vi "NI-9213_SoftPanel.vi"(3 "NI-9213 in Slot:":string="1") -> ()   [LabVIEW 2016]
uses:
  HelperSubVIs/GlobalControlVariables.vi
  <vilib>/Utility/TradDaqScaling.llb/Convert Thermocouple Reading (scaler).vi
panel:
  in  "Temperature Units":string(combo)="0"
  in  "TC 15 Type":string(combo)="0"
  in  "TC 14 Type":string(combo)="0"
  in  "TC 13 Type":string(combo)="0"
  in  "TC 12 Type":string(combo)="0"
  in  "TC 11 Type":string(combo)="0"
  in  "TC 10 Type":string(combo)="0"
  in  "TC 09 Type":string(combo)="0"
  in  "TC 08 Type":string(combo)="0"
  in  "TC 07 Type":string(combo)="0"
  in  "TC 06 Type":string(combo)="0"
  in  "TC 05 Type":string(combo)="0"
  in  "TC 04 Type":string(combo)="0"
  in  "TC 03 Type":string(combo)="0"
  in  "TC 02 Type":string(combo)="0"
  in  "TC 01 Type":string(combo)="0"
  in  "TC 00 Type":string(combo)="0"
  out "AI Values":sgl[](array[numeric])
  out "ExitModule":bool=TRUE
  out "TC 07":sgl
  out "TC 06":sgl
  out "TC 05":sgl
  out "TC 04":sgl
  out "TC 03":sgl
  out "TC 02":sgl
  out "TC 01":sgl
  out "TC 00":sgl
  out "TC 15":sgl min=0 max=5
  out "TC 14":sgl min=0 max=5
  out "TC 13":sgl min=0 max=5
  out "TC 12":sgl min=0 max=5
  out "TC 11":sgl min=0 max=5
  out "TC 10":sgl min=0 max=5
  out "TC 09":sgl min=0 max=5
  out "TC 08":sgl min=0 max=5
  in  "ExitButton":bool
  # "Thermocouple Type"
  # "Thermocouple Value"
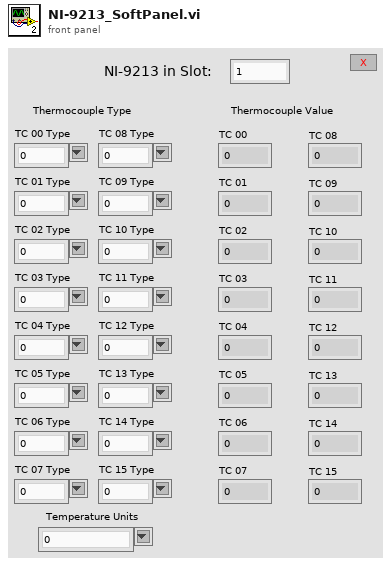
[diagram p1: front panel]
types:
  T1 = cluster{"[0]":sgl, "[1]":sgl, "[2]":sgl, "[3]":sgl, "[4]":sgl, "[5]":sgl, "[6]":sgl, "[7]":sgl, "[8]":sgl, "[9]":sgl, "[10]":sgl, "[11]":sgl, "[12]":sgl, "[13]":sgl, "[14]":sgl, "[15]":sgl}
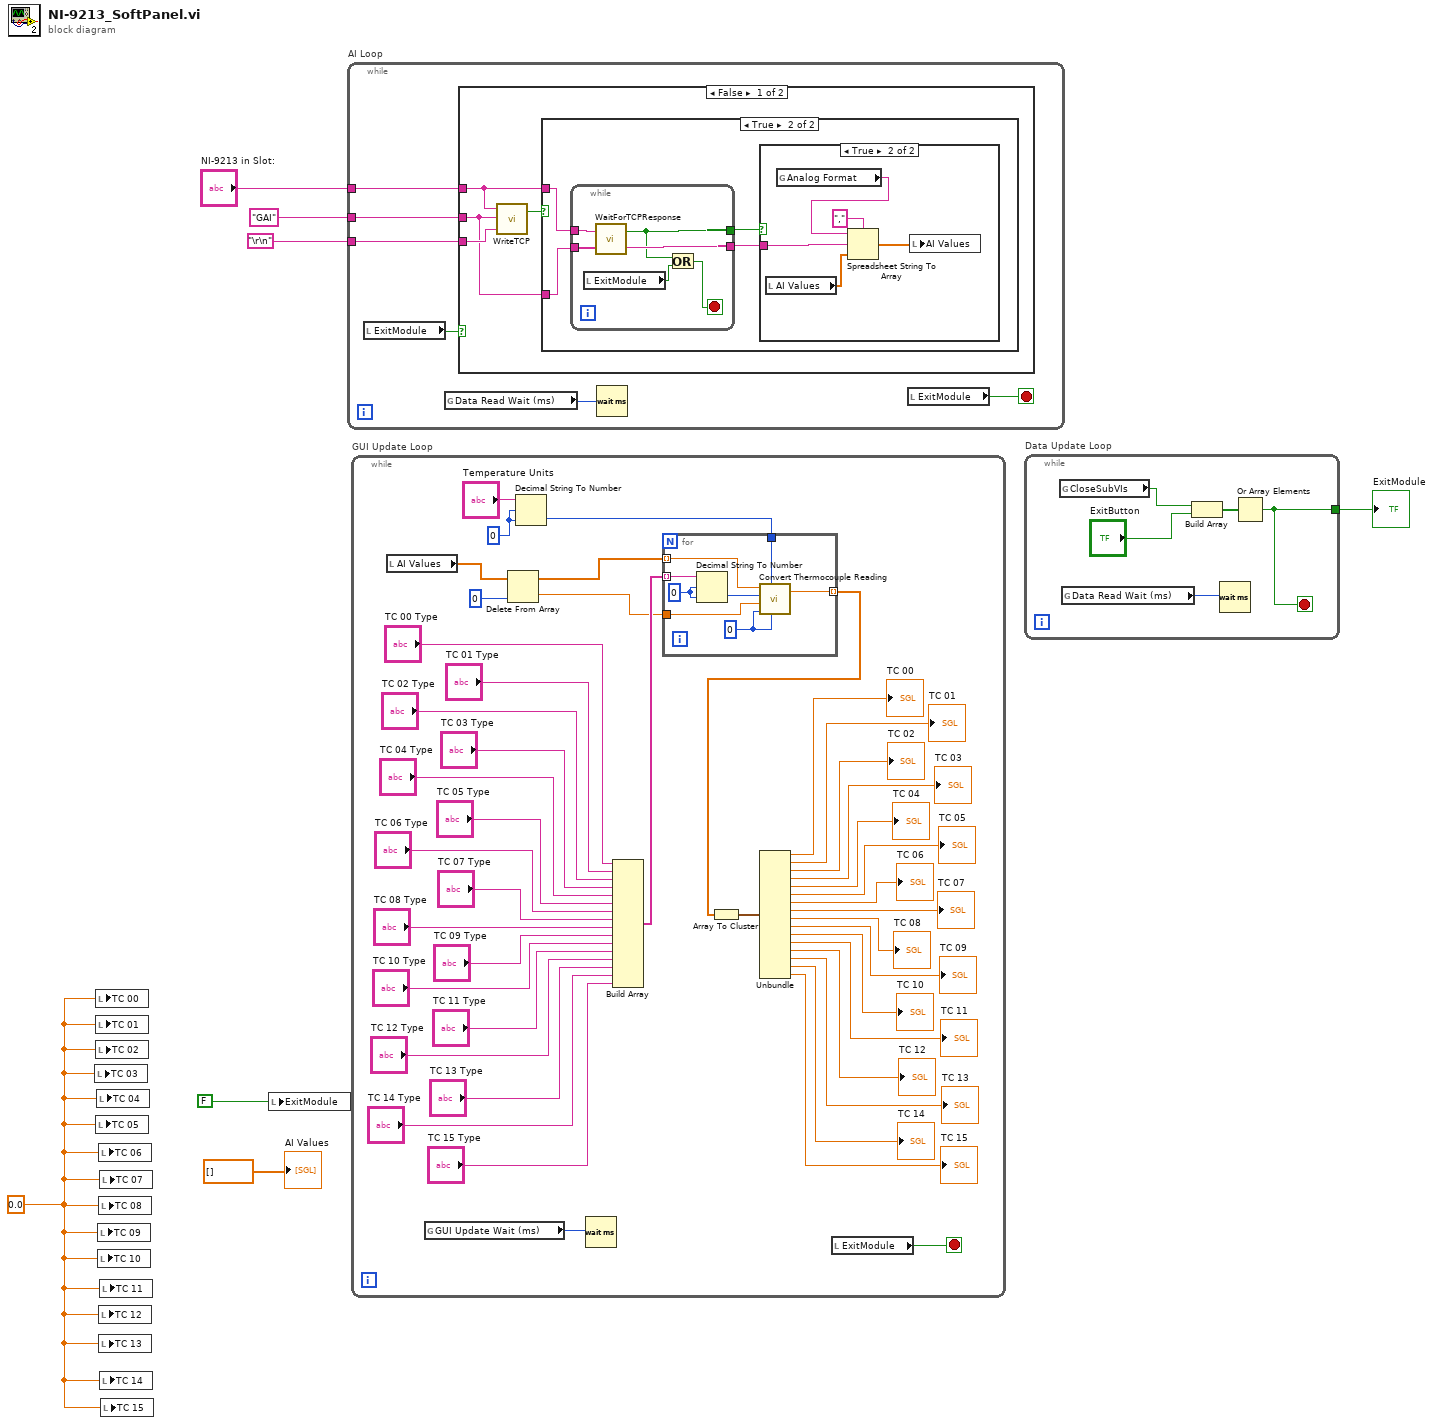
[diagram p0: block diagram]
diagram:
  w2 = 0.0
  n1 = local write "TC 03"(w2) -> ()
  n2 = local write "TC 00"(w2) -> ()
  n3 = local write "TC 01"(w2) -> ()
  n4 = local write "TC 02"(w2) -> ()
  n5 = local write "TC 05"(w2) -> ()
  n6 = local write "TC 04"(w2) -> ()
  n7 = local write "TC 09"(w2) -> ()
  n8 = local write "TC 10"(w2) -> ()
  n9 = local write "TC 06"(w2) -> ()
  n10 = local write "TC 08"(w2) -> ()
  n11 = local write "TC 12"(w2) -> ()
  n12 = local write "TC 13"(w2) -> ()
  n13 = local write "TC 07"(w2) -> ()
  n14 = local write "TC 11"(w2) -> ()
  n15 = local write "TC 14"(w2) -> ()
  n16 = local write "TC 15"(w2) -> ()
  n17 = local write "ExitModule"(FALSE) -> ()
  n18 = while "AI Loop" {
    tunnel: "NI-9213 in Slot:" -> [w12]
    tunnel: "\r\n" -> [w10]
    tunnel: "GAI" -> [w9]
    stop <- w13 stop-if-true
    n19 = local read "ExitModule"() -> (w8:bool)
    n20 = global read "GlobalControlVariables.vi" "Data Read Wait (ms)"() -> (w11:u32)
    n21 = case shown="False" w8 {
      tunnel: w12 -> [w16 _]
      tunnel: w10 -> [w15 _]
      tunnel: w9 -> [w14 _]
      frame False {
        n22 = call "WriteTCP.vi"("Data"=w15, "Action"=w14, "Module Slot"=w16) -> ("Sent"=w17:bool)  [unwired: 1 out]
        n23 = case shown="True" w17 {
          tunnel: w16 -> [_ w20]
          tunnel: w14 -> [_ w19]
          frame False {
          }
          frame True {
            n24 = while {
              tunnel: [w22] -> w21
              tunnel: w20 -> [w27]
              tunnel: w19 -> [w26]
              tunnel: [w25] -> w18
              stop <- w23 stop-if-true
              n25 = local read "ExitModule"() -> (w24:bool)
              n26 = call "WaitForTCPResponse.vi"("Action"=w26, "Module Slot"=w27) -> ("Received Data"=w25:string, "Ready"=w22:bool)
              n27 = Or(x=w22, y=w24) -> (x .or. y?=w23:bool)
            }
            n28 = case shown="True" w21 {
              tunnel: w18 -> [_ w32]
              frame False {
              }
              frame True {
                n29 = local read "AI Values"() -> (w28:sgl[])
                n30 = global read "GlobalControlVariables.vi" "Analog Format"() -> (w30:string)
                n31 = Spreadsheet String To Array(delimiter (Tab)=",", format string=w30, spreadsheet string=w32, array type (2D Dbl)=w28) -> (array=w29:sgl[])
                n32 = local write "AI Values"(w29) -> ()
              }
            }
          }
        }
      }
      frame True {
      }
    }
    n33 = Wait (ms)(milliseconds to wait=w11) -> ()  [unwired: 1 out]
    n34 = local read "ExitModule"() -> (w13:bool)
  }
  n35 = while "GUI Update Loop" {
    stop <- w74 stop-if-true
    w73 = u16 0
    n36 = local read "AI Values"() -> (w36:sgl[])
    n37 = global read "GlobalControlVariables.vi" "GUI Update Wait (ms)"() -> (w76:u32)
    n38 = Delete From Array(array=w36, index=u16 0) -> (deleted portion=w34:sgl, array with subset deleted=w35:sgl[])  [unwired: 1 in]
    n39 = Decimal String To Number(string="Temperature Units", offset=w73, default (0L)=w73) -> (number=w37:u16)  [unwired: 1 out]
    n40 = Wait (ms)(milliseconds to wait=w76) -> ()  [unwired: 1 out]
    n41 = Build Array("TC 00 Type", "TC 01 Type", "TC 02 Type", "TC 03 Type", "TC 04 Type", "TC 05 Type", "TC 06 Type", "TC 07 Type", "TC 08 Type", "TC 09 Type", "TC 10 Type", "TC 11 Type", "TC 12 Type", "TC 13 Type", "TC 14 Type", "TC 15 Type") -> (w39:string[])
    n42 = for {
      tunnel: w39 -> [w83] mode=indexing
      tunnel: w35 -> [w79] mode=indexing
      tunnel: w37 -> [w82]
      tunnel: [w81] -> w38 mode=indexing
      tunnel: w34 -> [w77]
      w78 = u16 0
      w84 = u16 0
      n43 = Decimal String To Number(string=w83, offset=w84, default (0L)=w84) -> (number=w80:u16)  [unwired: 1 out]
      n44 = call-poly <vilib>:"Convert Thermocouple Reading.vi"("Type of Excitation"=w78, "Temperature Units (C)"=w82, "CJC Sensor(0)"=w78, "CJC Voltage"=w77, "ThermocoupleType"=w80, "Thermocouple Voltage"=w79) -> ("Linearized Temperature"=w81:sgl)  [unwired: 1 in]
    }
    n45 = Array To Cluster(array=w38) -> (cluster=w75:T1)
    n46 = Unbundle(w75) -> ("[0]"=→"TC 00":sgl, "[1]"=→"TC 01":sgl, "[2]"=→"TC 02":sgl, "[3]"=→"TC 03":sgl, "[4]"=→"TC 04":sgl, "[5]"=→"TC 05":sgl, "[6]"=→"TC 06":sgl, "[7]"=→"TC 07":sgl, "[8]"=→"TC 08":sgl, "[9]"=→"TC 09":sgl, "[10]"=→"TC 10":sgl, "[11]"=→"TC 11":sgl, "[12]"=→"TC 12":sgl, "[13]"=→"TC 13":sgl, "[14]"=→"TC 14":sgl, "[15]"=→"TC 15":sgl)
    n47 = local read "ExitModule"() -> (w74:bool)
  }
  n48 = while "Data Update Loop" {
    tunnel: [w85] -> w7
    stop <- w85 stop-if-true
    n49 = global read "GlobalControlVariables.vi" "CloseSubVIs"() -> (w86:bool)
    n50 = global read "GlobalControlVariables.vi" "Data Read Wait (ms)"() -> (w89:u32)
    n51 = Build Array(w86, "ExitButton") -> (w88:bool[])
    n52 = Wait (ms)(milliseconds to wait=w89) -> ()  [unwired: 1 out]
    n53 = Or Array Elements(Boolean array=w88) -> (logical OR=w85:bool)
  }
  "ExitModule" <- w7
  "AI Values" <- sgl[] []
